vi "PanelFactory.vi"(8 "error in (no error)":errorcluster, 10 "ThreadName(\"\")":string, 11 "Admin_Actor in":refnum<class "Admin_Actor.lvclass">) -> (0 "error out":errorcluster, 2 "MemberPanel(Product)":refnum<class "MemberPanel.lvclass">, 3 "Admin_Actor out":refnum<class "Admin_Actor.lvclass">)   [LabVIEW 2015, in "Admin_Actor.lvlib" / "Admin_Actor.lvclass"]
uses:
  Admin_Actor.lvclass
  Member_Actor/MemberPanel/MemberPanel.lvclass
  ExcuseNotes/ExcuseNotesHandler.lvclass
  Admin_Actor.lvclass/Admin_Actor.ctl
  ExcuseNotes/ExcuseNotesHandler.lvclass/ExcuseNotesHandler.ctl
  CalAttendance/CalAttendance.lvclass
  <vilib>/Utility/error.llb/Error Cluster From Error Code.vi
  <vilib>/ErrorRing/Error Ring.xnode
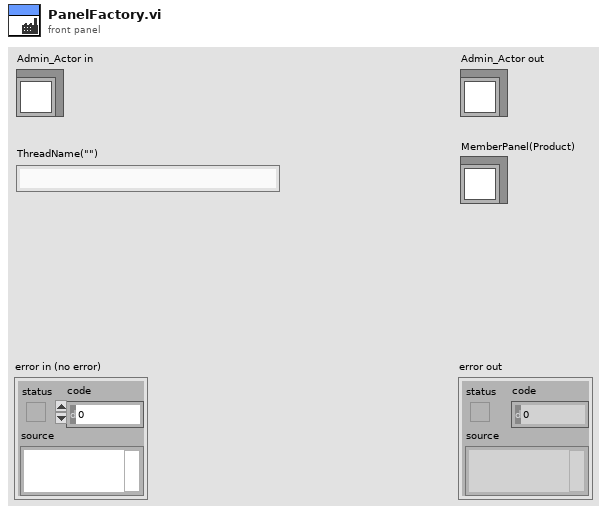
[diagram p1: front panel]
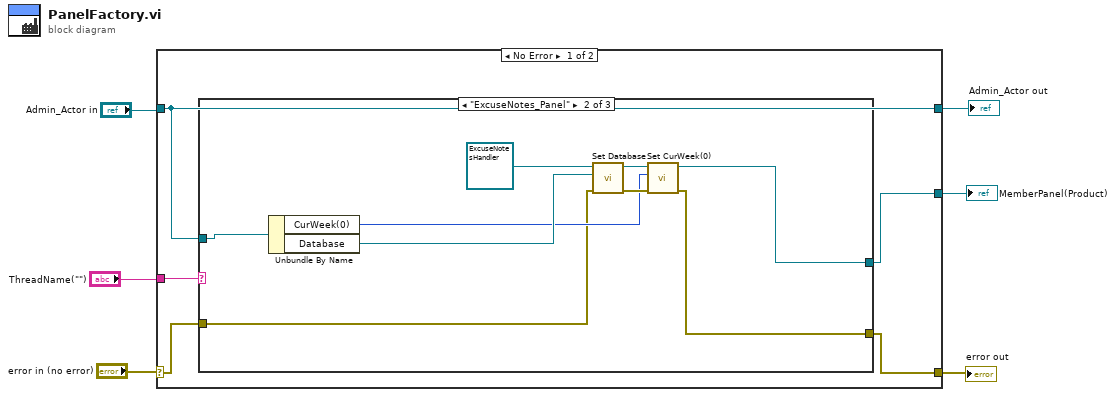
[diagram p0: block diagram]
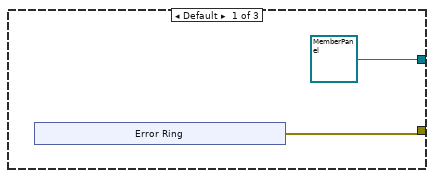
[diagram p2: hidden frame]
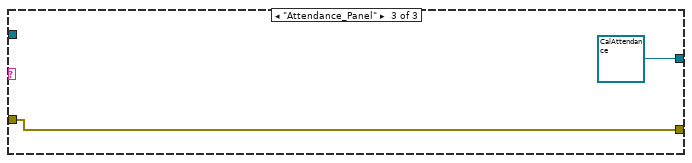
[diagram p3: hidden frame]
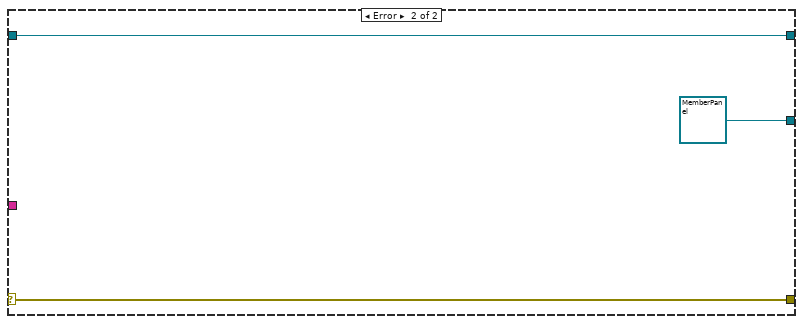
[diagram p4: hidden frame]
diagram:
  n1 = case shown="No Error" "error in (no error)" {
    selector: "error in (no error)" -> [w10 w32]
    tunnel: [w9 w32] -> w3
    tunnel: [w8 w31] -> w4
    tunnel: "Admin_Actor in" -> [w8 w31]
    tunnel: "ThreadName(\"\")" -> [w11 _]
    tunnel: [w7 refnum<class "MemberPanel.lvclass"> refnum ("MemberInfo out")] -> w2
    frame No Error {
      n2 = case shown="\"ExcuseNotes_Panel\"" w11 {
        tunnel: w10 -> [_ w21 w29]
        tunnel: [w12 w20 w29] -> w9
        tunnel: w8 -> [_ w27 _]
        tunnel: [refnum<class "MemberPanel.lvclass"> refnum ("MemberInfo out") w19 refnum<class "CalAttendance.lvclass"> refnum ("Admin_Actor.lvlib:CalAttendance")] -> w7
        frame Default {
          n3 = xnode "Error Ring"() -> ("error out"=w12:errorcluster)
        }
        frame "ExcuseNotes_Panel" {
          n4 = Unbundle By Name(w27) -> ("CurWeek(0)"=w22:i32, "Database"=w23:refnum<class "Database.lvclass">)
          n5 = call "Set Database.vi"("error in (no error)"=w21, "Database"=w23, "ExcuseNotes in"=refnum<class "ExcuseNotesHandler.lvclass"> refnum ("Admin_Actor.lvlib:ExcuseNotes.lvclass")) -> ("error out"=w26:errorcluster, "ExcuseNotes out"=w25:refnum<class "ExcuseNotesHandler.lvclass">)  [unwired: 7 in]
          n6 = call "Set CurWeek(0).vi"("error in (no error)"=w26, "CurWeek(0)"=w22, "ExcuseNotesHandler in"=w25) -> ("error out"=w20:errorcluster, "ExcuseNotesHandler out"=w19:refnum<class "ExcuseNotesHandler.lvclass">)  [unwired: 7 in]
        }
        frame "Attendance_Panel" {
        }
      }
    }
    frame Error {
    }
  }
  "error out" <- w3
  "Admin_Actor out" <- w4
  "MemberPanel(Product)" <- w2
